vi "ver1.vi"() -> ()   [LabVIEW 2010]
panel:
  in  "2 y 2":dbl
  in  "1 y 2":dbl
  in  "2 x 2":dbl
  in  "1 x 2":dbl
  in  "2nm 2":dbl
  in  "Array":dbl[](array[numeric])
  in  "zero nm":dbl
  in  "stop":bool
  out "x out":dbl
  out "y out":dbl
  in  "nm in":dbl
  in  "y in":dbl
  in  "x in":dbl
  in  "Volts/pixel":dbl
  in  "2 y":dbl
  in  "1 y":dbl
  in  "2 x":dbl
  in  "1 x":dbl
  in  "2nm":dbl
  in  "1nm":dbl
  # "x"
  # "y"
  # "Wavelength"
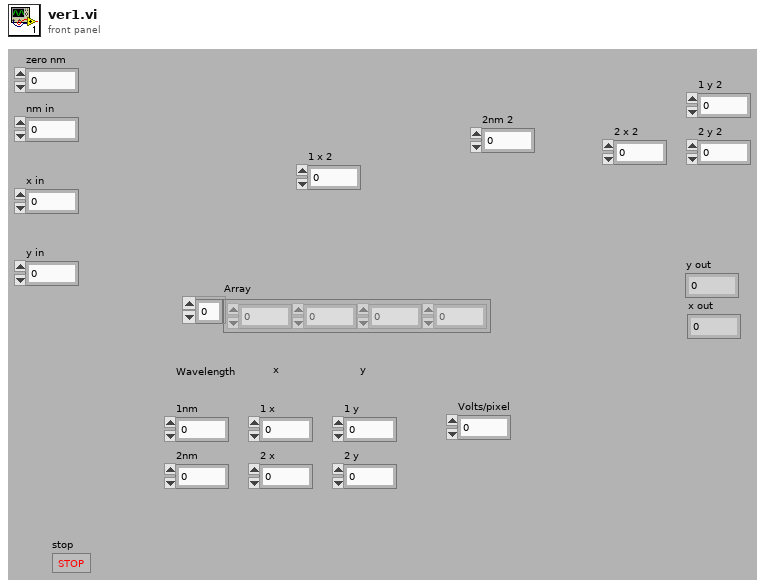
[diagram p1: front panel]
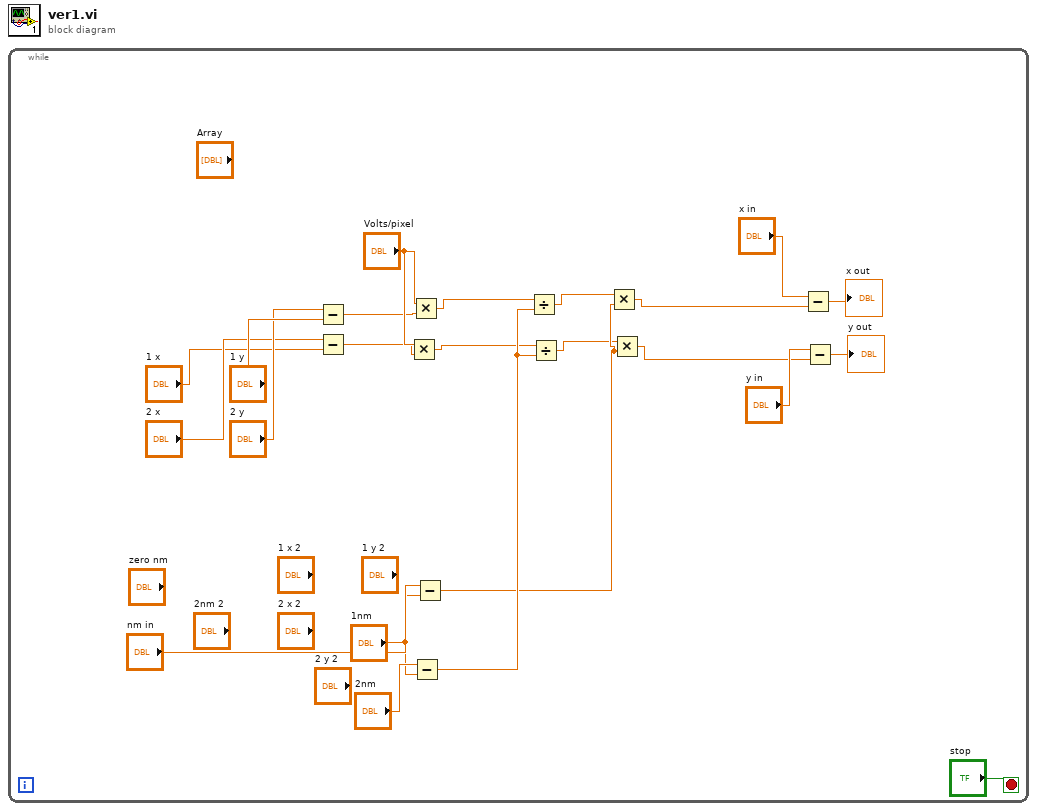
[diagram p0: block diagram]
diagram:
  n1 = while {
    stop <- "stop" stop-if-true
    n2 = Subtract(x="2 y", y="1 y") -> (x-y=w22:dbl)
    n3 = Subtract(x="2 x", y="1 x") -> (x-y=w21:dbl)
    n4 = Multiply(x="Volts/pixel", y=w21) -> (x*y=w15:dbl)
    n5 = Multiply(x="Volts/pixel", y=w22) -> (x*y=w14:dbl)
    n6 = Subtract(x="2nm", y="1nm") -> (x-y=w16:dbl)
    n7 = Subtract(x="nm in", y="1nm") -> (x-y=w11:dbl)
    n8 = Divide(x=w14, y=w16) -> (x/y=w10:dbl)
    n9 = Divide(x=w15, y=w16) -> (x/y=w9:dbl)
    n10 = Multiply(x=w10, y=w11) -> (x*y=w8:dbl)
    n11 = Multiply(x=w9, y=w11) -> (x*y=w6:dbl)
    n12 = Subtract(x="x in", y=w8) -> (x-y=→"x out":dbl)
    n13 = Subtract(x="y in", y=w6) -> (x-y=→"y out":dbl)
  }
